vi "Convert TDMS to CSV.vi"(8 "error in (no error)":errorcluster, 10 "CSV Settings":T1={"Log Stats"=FALSE, "Time Format"="%H:%M:%S%3u", "Resampled"=FALSE, "Resampled Rate"=0.0, "Digits of Precision"=0, "Relative Time"=FALSE, "Log Units"=FALSE, "Log Properties"=FALSE}, 11 "TDMS File":path) -> (0 "error out":errorcluster)   [LabVIEW 2022 SP3, in "CSV Export.lvlib" / "CSV Export.lvclass"]
uses:
  CSV Export.lvclass
  Controls/CSV Export Settings.ctl
  <vilib>/measure/maresamp.llb/Resample N Waveforms (continuous, t0 DBL).vi
  CSV Export.lvclass/CSV Export.ctl
  <vilib>/measure/NI_MAPro.lvlib
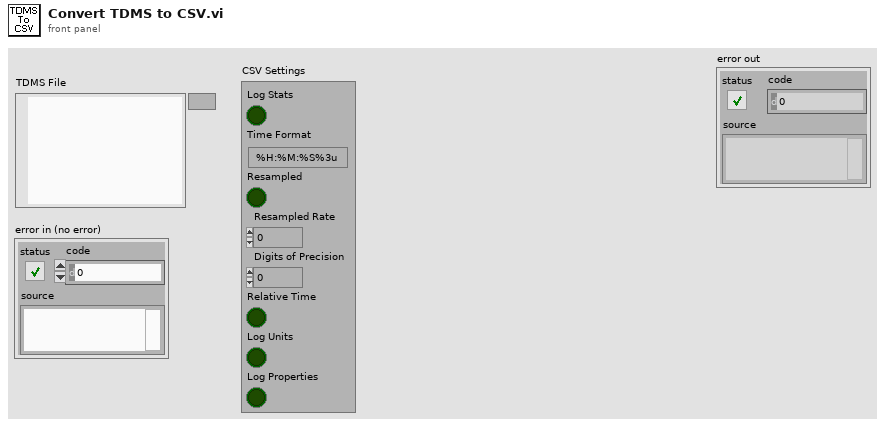
[diagram p1: front panel]
types:
  T1 = typedef "CSV Export.lvlib/CSV Export.lvclass/CSV Export Settings.ctl" = cluster{"Log Stats":bool, "Time Format":string, "Resampled":bool, "Resampled Rate":dbl, "Digits of Precision":u32, "Relative Time":bool, "Log Units":bool, "Log Properties":bool}
  T2 = cluster{"tdms file out":refnum<k34>, "group name out":string, string}
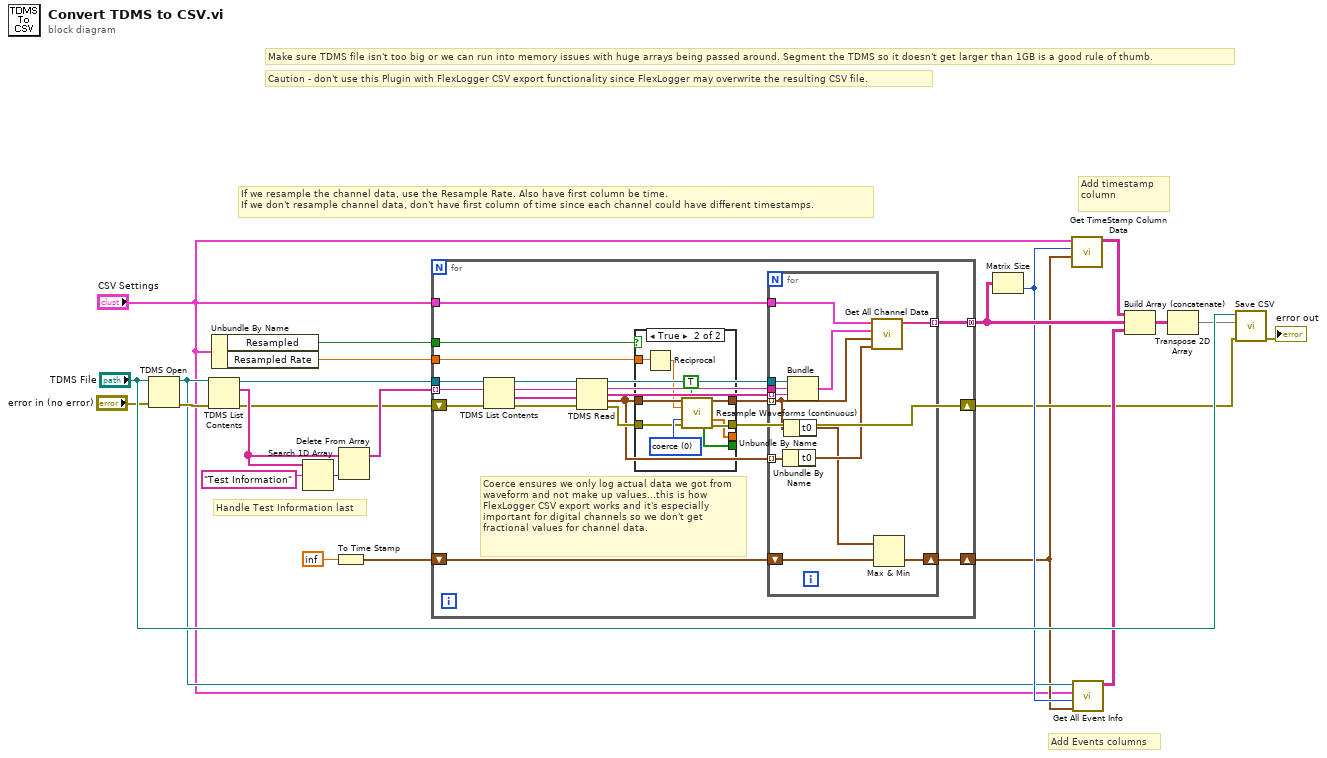
[diagram p0: block diagram]
diagram:
  # "Add Events columns"
  # "Make sure TDMS file isn't too big or we can run into memory issues with huge arrays being passed around. Segment the TDMS so it doesn't get larger than 1GB is a good rule of thumb."
  # "Caution - don't use this Plugin with FlexLogger CSV export functionality since FlexLogger may overwrite the resulting CSV file."
  # "Add timestamp column"
  # "If we resample the channel data, use the Resample Rate. Also have first column be time.\nIf we don't resample channel data, don't have first column of time since each channel could have different timestamps."
  # "Handle Test Information last"
  n1 = TDMS Open(8:"error in (no error)", 11:"TDMS File") -> (0:w24:errorcluster, 3:w8:refnum<k34>)  [unwired: 5 in]
  n2 = TDMS List Contents(4:w24, 7:w8) -> (0:w19:errorcluster, 2:w22:string[], 3:w11:refnum<k34>)  [unwired: 1 in, 1 out]
  n3 = Unbundle By Name("CSV Settings") -> ("Resampled"=w18:bool, "Resampled Rate"=w17:dbl)
  n4 = Search 1D Array(1D array=w22, element="Test Information" ("group name")) -> (index of element=w21:i32)  [unwired: 1 in]
  n5 = To Time Stamp(1:inf) -> (0:w15:timestamp)
  n6 = Delete From Array(array=w22, index=w21) -> (array with subset deleted=w20:string[])  [unwired: 1 in, 1 out]
  n7 = for {
    tunnel: w20 -> [w43] mode=indexing
    tunnel: w11 -> [w44]
    tunnel: w18 -> [w35]
    tunnel: w17 -> [w38]
    shift-right: [w33] -> w4
    shift-left: w15 -> [w34]
    tunnel: [w32] -> w14 mode=concatenating
    shift-right: [w31] -> w7
    shift-left: w19 -> [w39]
    tunnel: "CSV Settings" -> [w25]
    # "Coerce ensures we only log actual data we got from waveform and not make up values...this is how FlexLogger CSV export works and it's especially important for digital channels so we don't get fractional values for channel data."
    n8 = TDMS List Contents(4:w39, 6:w43, 7:w44) -> (0:w40:errorcluster, 1:w27:string[], 2:w28:string, 3:w29:refnum<k34>)
    n9 = TDMS Read(0:w29, 5:w28, 7:w27, 11:w40) -> (4:w26:refnum<k34>, 6:w41:string, 8:w42:string[], 10:w30:waveform(dbl)[], 15:w37:errorcluster)  [unwired: 4 in, 1 out]
    n10 = case shown="True" w35 {
      tunnel: w30 -> [w46 w56]
      tunnel: w38 -> [_ w53]
      tunnel: w37 -> [w45 w51]
      tunnel: [w46 w50] -> w36
      tunnel: [w45 w49] -> w31
      tunnel: [_ w48] -> _
      tunnel: [_ w47] -> _
      frame False {
      }
      frame True {
        w55 = u16 0 items=["coerce", "linear", "spline", "FIR filter"] ("interpolation mode")
        n11 = Reciprocal(x=w53) -> (1/x=w52:dbl)
        n12 = call-poly <vilib>:"Resample Waveforms (continuous).vi"("waveforms in"=w56, "reset"=TRUE, "dt"=w52, "interpolation mode"=w55, "error in (no error)"=w51) -> ("resampled waveforms out"=w50:waveform(dbl)[], "used t0's"=w47:dbl[], "t0 adjusted warnings"=w48:bool[], "error out"=w49:errorcluster)  [unwired: 6 in, 1 out]
      }
    }
    n13 = for {
      tunnel: w36 -> [w58] mode=indexing
      tunnel: w42 -> [w63] mode=indexing
      tunnel: w41 -> [w64]
      shift-right: [w67] -> w33
      shift-left: w34 -> [w68]
      tunnel: [w59] -> w32 mode=indexing
      tunnel: w30 -> [w66] mode=indexing
      tunnel: w26 -> [w65]
      tunnel: w25 -> [w62]
      n14 = Unbundle By Name(w66) -> ("t0"=w60:timestamp)
      n15 = Unbundle By Name(w58) -> ("t0"=w57:timestamp)
      n16 = Bundle("tdms file out"=w65, "group name out"=w64, w63) -> (w61:T2)  [unwired: 1 in]
      n17 = call "Get All Channel Data.vi"("Original T0"=w60, "waveform in"=w58, "TDMS Channel Info"=w61, "CSV Settings"=w62) -> ("String Data"=w59:string[])  [unwired: 7 in]
      n18 = Max & Min(x=w57, y=w68) -> (min(x,y)=w67:timestamp)  [unwired: 1 out]
    }
  }
  n19 = Matrix Size(0:w14) -> (2:w9:i32)  [unwired: 1 out]
  n20 = call "Get TimeStamp Column Data.vi"("First T0"=w4, "Array Size"=w9, "CSV Settings"="CSV Settings") -> ("Timestamp Column Data"=w1:string[][])  [unwired: 8 in]
  n21 = call "Get All Event Info.vi"("First T0"=w4, "Array Size"=w9, "CSV Settings"="CSV Settings", "Tdms File Ref In"=w8) -> ("Test Info Column Data"=w10:string[][])  [unwired: 7 in]
  n22 = Build Array (concatenate)(w1, w14, w10) -> (w13:string[][])
  n23 = Transpose 2D Array(2D array=w13) -> (transposed array=w2:string[][])
  n24 = call "Save CSV.vi"("error in"=w7, "CSV Data"=w2, "TDMS File"="TDMS File") -> ("error out"=→"error out":errorcluster)  [unwired: 8 in]
